vi "MT Generate FSK System Parameters(M).vi"(0 "samples per symbol (16)":i32=16, 5 "M-FSK (2)":i32=2, 7 "FSK deviation (Hz)":dbl=150000.0 format="%.2p", 9 "symbol phase continuity":enum16{"continuous", "discontinuous"}(ring), 11 "error in (no error)":errorcluster) -> (6 "FSK system parameters":T1 {"symbol map" format="%.2f"}, 8 "bits per symbol":i32, 15 "error out":errorcluster)   [LabVIEW 2020, in "niDMT.lvlib"]
doc: "This polymorphic instance calculates parameters for use with either the MT Modulate FSK or MT Demodulate FSK VI. This VI generates the symbol map for FSK-modulated systems. This VI accepts an M-ary value that specifies a predefined symbol map with the number of distinct symbol map values to use as symbols."
uses:
  <vilib>/addons/Modulation/niDMT.lvlib
  <vilib>/addons/Modulation/Digital/Support/Controls/FSK System Parameters.ctl
  <vilib>/Analysis/1siggen.llb/Ramp Pattern by Samples.vi
  <vilib>/addons/Modulation/niAMT.lvlib
  <vilib>/Analysis/NI_AALBase.lvlib
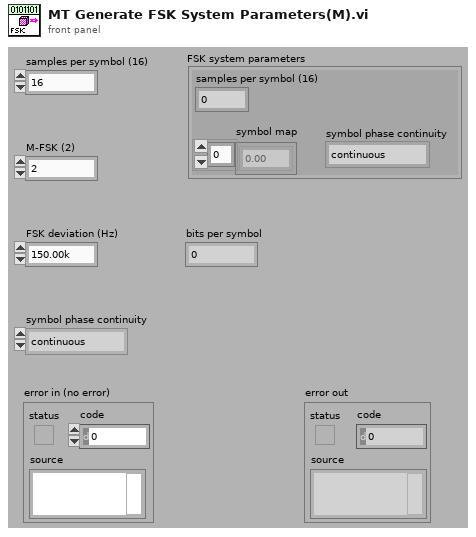
[diagram p1: front panel]
types:
  T1 = cluster{"samples per symbol (16)":i32, "symbol map":dbl[], "symbol phase continuity":enum16{"continuous", "discontinuous"}}
  T2 = typedef "niDMT.lvlib/FSK System Parameters.ctl" = cluster{"samples per symbol (16)":i32, "symbol map":dbl[], "symbol phase continuity":enum16{"continuous", "discontinuous"}}
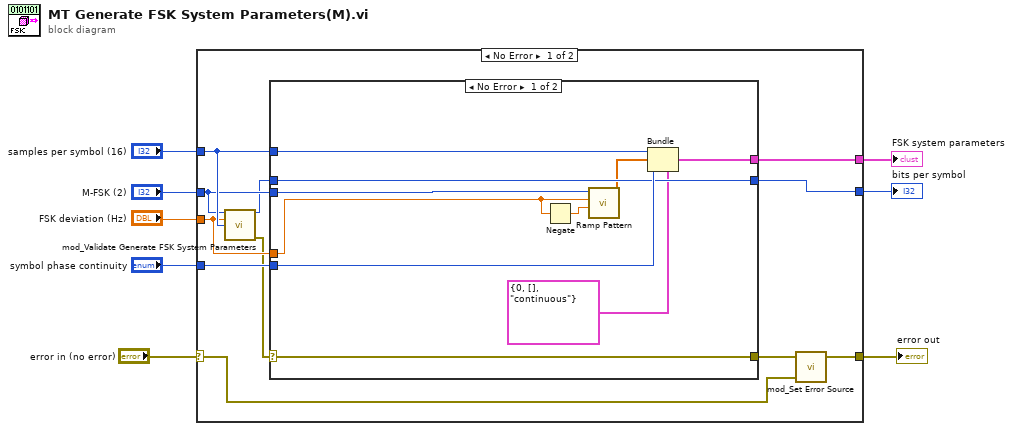
[diagram p0: block diagram]
diagram:
  n1 = case shown="No Error" "error in (no error)" {
    selector: "error in (no error)" -> [w15 w31]
    tunnel: "samples per symbol (16)" -> [w13 _]
    tunnel: "symbol phase continuity" -> [w19 _]
    tunnel: "M-FSK (2)" -> [w11 _]
    tunnel: [w18 _] -> w5
    tunnel: "FSK deviation (Hz)" -> [w12 _]
    tunnel: [w17 _] -> w3
    tunnel: [w16 w31] -> w1
    frame No Error {
      n2 = call <vilib>:"mod_Validate Generate FSK System Parameters.vi"("M-FSK"=w11, "deviation"=w12, "samples per symbol"=w13) -> ("bits per symbol"=w9:i32, "error out"=w10:errorcluster)  [unwired: 11 out]
      n3 = case shown="No Error" w10 {
        selector: w10 -> [w20 w30]
        tunnel: w13 -> [w29 _]
        tunnel: w19 -> [w28 _]
        tunnel: w11 -> [w27 _]
        tunnel: [w26 _] -> w18
        tunnel: w12 -> [w25 _]
        tunnel: [w24 _] -> w17
        tunnel: [w20 w30] -> w14
        tunnel: w9 -> [w24 _]
        frame No Error {
          n4 = Negate(x=w25) -> (-x=w23:dbl)
          n5 = call-poly <vilib>:"Ramp Pattern.vi"("start"=w23, "end"=w25, "samples"=w27) -> ("Ramp Pattern"=w22:dbl[])  [unwired: 7 in, 1 out]
          n6 = Bundle(cluster=T2 {"samples per symbol (16)"=0, "symbol map"=[], "symbol phase continuity"=enum."continuous"} ("FSK system parameters"), "samples per symbol (16)"=w29, "symbol map"=w22, "symbol phase continuity"=w28) -> (w26:T2)
        }
        frame Error {
        }
      }
      n7 = call <vilib>:"mod_Set Error Source.vi"("initial error in (no error)"=w15, "final error in (no error)"=w14) -> ("error out"=w16:errorcluster)  [unwired: 3 out]
    }
    frame Error {
    }
  }
  "FSK system parameters" <- w5
  "bits per symbol" <- w3
  "error out" <- w1
